vi "Set Calculation State.vi"(8 "error in (no error)":errorcluster, 10 "Continuous":bool, 11 "CPU FFT Calculator in":refnum<class "CPU FFT Calculator.lvclass">) -> (0 "error out":errorcluster, 3 "CPU FFT Calculator out":refnum<class "CPU FFT Calculator.lvclass">)   [LabVIEW 2020, in "CPU FFT Calculator.lvlib" / "CPU FFT Calculator.lvclass"]
uses:
  CPU FFT Calculator.lvclass
  Calculation Worker/Calculation Worker/Calculation Worker.lvclass
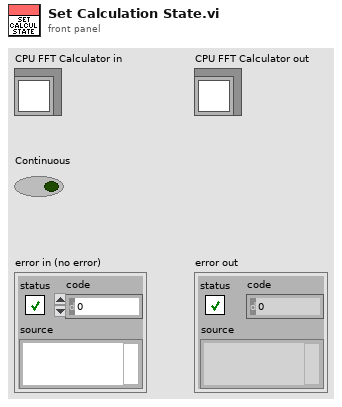
[diagram p1: front panel]
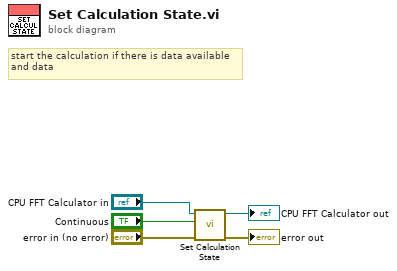
[diagram p0: block diagram]
diagram:
  # "start the calculation if there is data available\nand data"
  n1 = call-parent "Set Calculation State.vi"("error in (no error)"="error in (no error)", "Continuous"="Continuous", "Calculation Worker in"="CPU FFT Calculator in") -> ("error out"=→"error out":errorcluster, "Calculation Worker out"=→"CPU FFT Calculator out":refnum<class "CPU FFT Calculator.lvclass">)  [unwired: 7 in]
